vi "Evaluate In Range Trigger (Array).vi"(8 "error in (no error)":errorcluster, 10 "Trigger Data":dbl[](array[numeric]), 11 "In Range Trigger in":refnum<class "In Range Trigger.lvclass">) -> (0 "error out":errorcluster, 1 "Trigger indices":i32[](array[numeric]), 2 "Trigger":bool, 3 "In Range Trigger out":refnum<class "In Range Trigger.lvclass">)   [LabVIEW 2015, in "In Range Trigger.lvclass"]
uses:
  In Range Trigger.lvclass
  In Range Trigger.lvclass/In Range Trigger.ctl
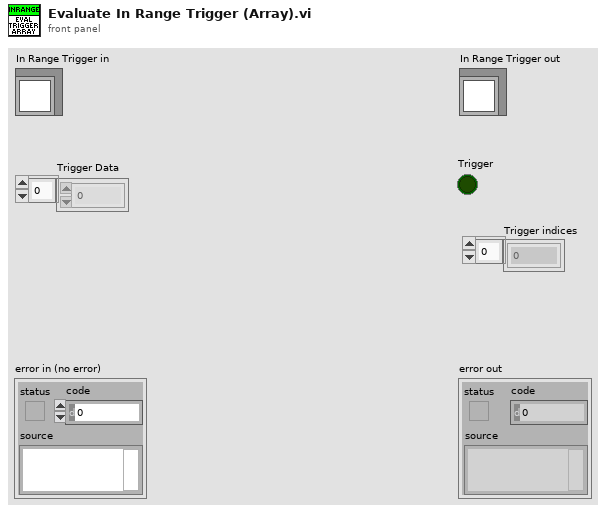
[diagram p1: front panel]
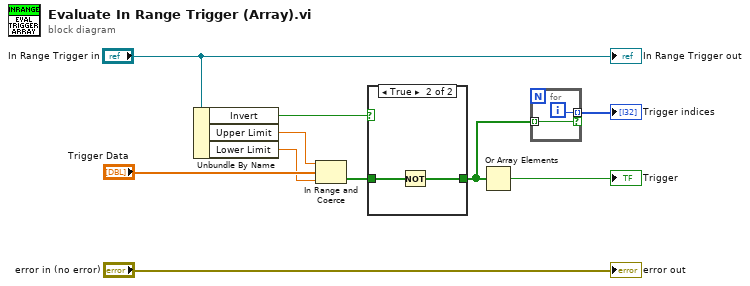
[diagram p0: block diagram]
diagram:
  n1 = Unbundle By Name("In Range Trigger in") -> ("Invert"=w5:bool, "Upper Limit"=w7:dbl, "Lower Limit"=w6:dbl)
  n2 = In Range and Coerce(upper limit=w7, x="Trigger Data", lower limit=w6) -> (In Range?=w4:bool[])  [unwired: 1 out]
  n3 = case shown="True" w5 {
    tunnel: [w11 w13] -> w1
    tunnel: w4 -> [w11 w12]
    frame False {
    }
    frame True {
      n4 = Not(x=w12) -> (.not. x?=w13:bool[])
    }
  }
  n5 = Or Array Elements(Boolean array=w1) -> (logical OR=→"Trigger":bool)
  n6 = for {
    tunnel: w1 -> [w14] mode=indexing
    tunnel: [w15] -> w2 mode=indexing if=w14
    i -> [w15]
  }
  "Trigger indices" <- w2
  "error out" <- "error in (no error)"
  "In Range Trigger out" <- "In Range Trigger in"
